vi "dfd_Bilinear Mapping.vi"(1 "s-plane poles/zeros":T1[](array[typedef])) -> (0 "z-plane poles/zeros":T1[](array[typedef]))   [LabVIEW 2017, in "NI_DigFilter_Design.lvlib"]
uses:
  <vilib>/addons/Digital Filter Design/NI_DigFilter_Design.lvlib
  <vilib>/addons/Digital Filter Design/_Objects.llb/DFD Pole-Zero.ctl
  <vilib>/addons/Digital Filter Design/NI_DigFilterLicensed.lvlib
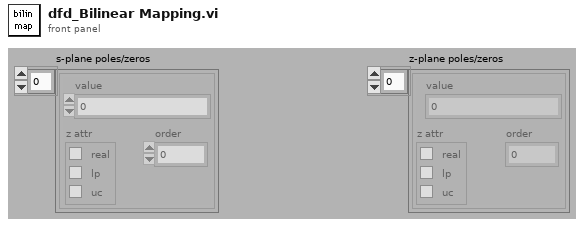
[diagram p1: front panel]
types:
  T1 = typedef "NI_DigFilterLicensed.lvlib/DFD Pole-Zero.ctl" = cluster{"value":cdb, "z attr":cluster{"real":bool, "lp":bool, "uc":bool}, "order":i32}
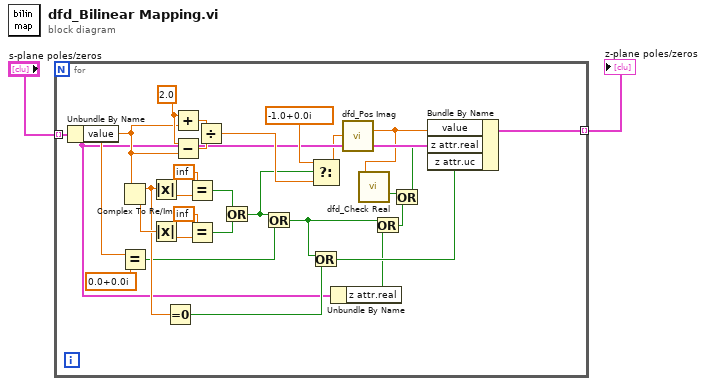
[diagram p0: block diagram]
diagram:
  n1 = for {
    tunnel: "s-plane poles/zeros" -> [w10] mode=indexing
    tunnel: [w18] -> w1 mode=indexing
    w19 = 2.0
    n2 = Unbundle By Name(w10) -> ("value"=w16:cdb)
    n3 = Complex To Re/Im(x + iy=w16) -> (x=w14:dbl, y=w26:dbl)
    n4 = Equal?(x=w16, y=cdb 0.0+0.0i) -> (x = y?=w12:bool)
    n5 = Absolute Value(x=w14) -> (abs(x)=w23:dbl)
    n6 = Absolute Value(x=w26) -> (abs(x)=w24:dbl)
    n7 = Equal To 0?(x=w14) -> (x = 0?=w13:bool)
    n8 = Add(x=w19, y=w16) -> (x+y=w20:cdb)
    n9 = Subtract(x=w19, y=w16) -> (x-y=w21:cdb)
    n10 = Equal?(x=inf, y=w23) -> (x = y?=w27:bool)
    n11 = Equal?(x=inf, y=w24) -> (x = y?=w28:bool)
    n12 = Divide(x=w20, y=w21) -> (x/y=w30:cdb)
    n13 = Or(x=w27, y=w28) -> (x .or. y?=w15:bool)
    n14 = Or(x=w15, y=w12) -> (x .or. y?=w9:bool)
    n15 = Select(t=cdb -1.0+0.0i, s=w15, f=w30) -> (s? t:f=w4:cdb)
    n16 = Or(x=w9, y=w13) -> (x .or. y?=w11:bool)
    n17 = Unbundle By Name(w10) -> ("z attr.real"=w8:bool)
    n18 = call <vilib>:"dfd_Pos Imag.vi"("complex in"=w4) -> ("complex out"=w3:cdb)
    n19 = call <vilib>:"dfd_Check Real.vi"("complex"=w3) -> ("real?"=w6:bool)
    n20 = Or(x=w9, y=w8) -> (x .or. y?=w7:bool)
    n21 = Or(x=w6, y=w7) -> (x .or. y?=w5:bool)
    n22 = Bundle By Name(cluster=w10, "value"=w3, "z attr.real"=w5, "z attr.uc"=w11) -> (w18:T1)
  }
  "z-plane poles/zeros" <- w1
